vi "Dispose.vi"(8 "error in (no error)":errorcluster, 11 "ProductB":refnum<class "ProductB.lvclass">) -> (0 "error out":errorcluster)   [LabVIEW 2020, in "FactoryMethod.lvlib" / "FactoryMethodLazyEvaluation.lvlib" / "ProductB.lvclass"]
uses:
  ProductB.lvclass
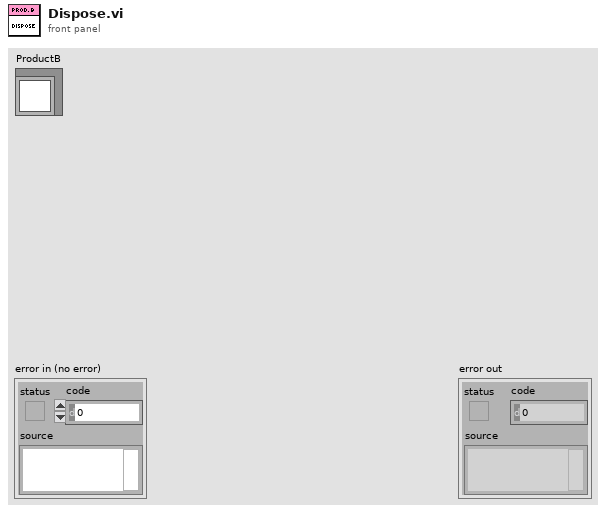
[diagram p1: front panel]
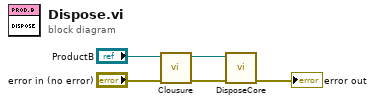
[diagram p0: block diagram]
diagram:
  n1 = call-dynamic "Clousure.vi"("error in (no error)"="error in (no error)", "ProductB"="ProductB") -> ("error out"=w3:errorcluster, "ProductB"=w1:refnum<class "ProductB.lvclass">)  [unwired: 8 in]
  n2 = call-dynamic "DisposeCore.vi"("error in (no error)"=w3, "ProductB"=w1) -> ("error out"=→"error out":errorcluster)  [unwired: 8 in, 1 out]
